vi "Delete_Zero_Columns_Rows_Resolved_Tracks-1.vi"(4 "error IN":errorcluster, 7 "[IN] Clusters for Re\nconstructed Tracks":T1) -> (0 "error OUT":errorcluster, 3 "[OUT] Clusters for Re\nconstructed Tracks":T1)   [LabVIEW 2013]
doc: "The subVI delete zero columns and rows after resolving the correspondence problems"
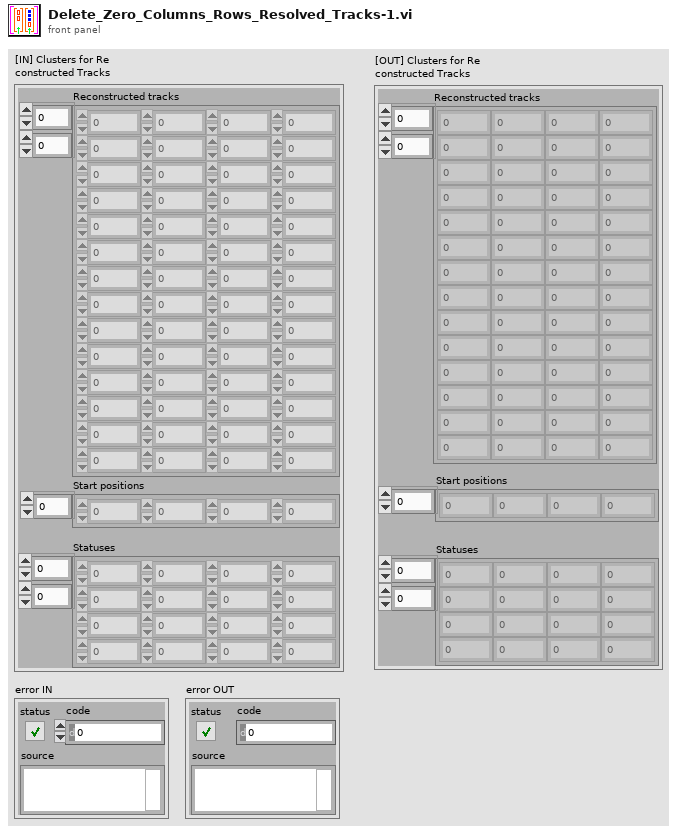
[diagram p1: front panel]
types:
  T1 = cluster{"Reconstructed tracks":dbl[][], "Start positions":i32[], "Statuses":i16[][]}
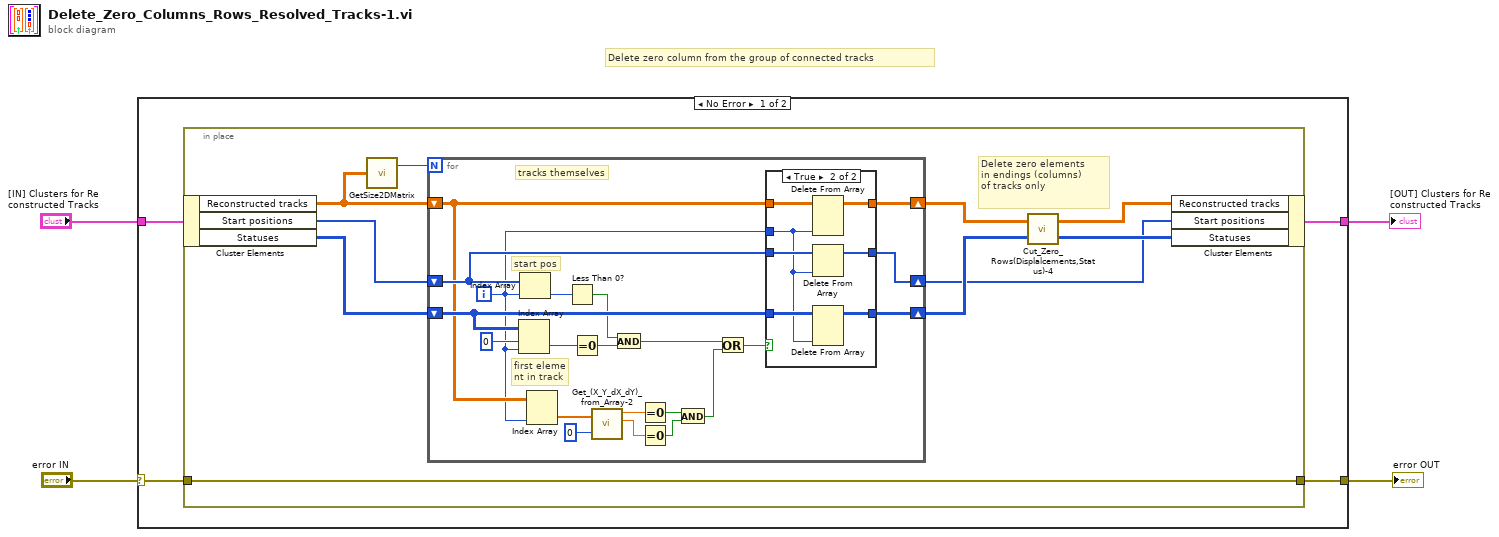
[diagram p0: block diagram]
diagram:
  # "Delete zero column from the group of connected tracks"
  n1 = case shown="No Error" "error IN" {
    selector: "error IN" -> [w6 w51]
    tunnel: "[IN] Clusters for Re\nconstructed Tracks" -> [w8 w50]
    tunnel: [w7 w50] -> w3
    tunnel: [w5 w51] -> w1
    frame No Error {
      n2 = in-place {
        in-place-border: w6 -> [w9]
        in-place-border: [w9] -> w5
        # "Delete zero elements \nin endings (columns)\nof tracks only"
        n3 = in-place-cluster #1(w8) -> ("Reconstructed tracks"=w15:dbl[][], "Start positions"=w11:i32[], "Statuses"=w10:i16[][])
        n4 = call "GetSize2DMatrix.vi"("Array IN (2D)"=w15) -> ("# Cols"=w18:i32)  [unwired: 1 out]
        n5 = for {
          N: w18 -> [_]
          shift-right: [w34] -> w17
          shift-left: w15 -> [w28]
          shift-right: [w33] -> w12
          shift-left: w11 -> [w36]
          shift-right: [w32] -> w16
          shift-left: w10 -> [w35]
          i -> [w27]
          # "tracks themselves"
          # "start pos"
          # "first eleme\nnt in track"
          n6 = Index Array(array=w35, index (row)=0, index (col)=w27) -> (element=w37:i16)
          n7 = Index Array(array=w36, index=w27) -> (element=w38:i32)
          n8 = Index Array(array=w28, index (col)=w27) -> (element=w26:dbl[])  [unwired: 1 in]
          n9 = Less Than 0?(x=w38) -> (x < 0?=w30:bool)
          n10 = Equal To 0?(x=w37) -> (x = 0?=w31:bool)
          n11 = call "Get_(X_Y_dX_dY)_from_Array-2.vi"("(X,Y,dX,dY)"=w26, "Index of Displacement"=0) -> ("X"=w24:dbl, "Y"=w23:dbl)  [unwired: 2 out]
          n12 = And(x=w30, y=w31) -> (x .and. y?=w29:bool)
          n13 = Equal To 0?(x=w24) -> (x = 0?=w22:bool)
          n14 = Equal To 0?(x=w23) -> (x = 0?=w21:bool)
          n15 = And(x=w22, y=w21) -> (x .and. y?=w19:bool)
          n16 = Or(x=w29, y=w19) -> (x .or. y?=w20:bool)
          n17 = case shown="True" w20 {
            tunnel: w28 -> [w42 w49]
            tunnel: w27 -> [_ w43]
            tunnel: w36 -> [w41 w48]
            tunnel: w35 -> [w40 w45]
            tunnel: [w42 w47] -> w34
            tunnel: [w41 w46] -> w33
            tunnel: [w40 w44] -> w32
            frame False {
            }
            frame True {
              n18 = Delete From Array(array=w49, index (col)=w43) -> (array with subset deleted=w47:dbl[][])  [unwired: 2 in, 1 out]
              n19 = Delete From Array(array=w48, index=w43) -> (array with subset deleted=w46:i32[])  [unwired: 1 in, 1 out]
              n20 = Delete From Array(array=w45, index (col)=w43) -> (array with subset deleted=w44:i16[][])  [unwired: 2 in, 1 out]
            }
          }
        }
        n21 = call "Cut_Zero_Rows(Displalcements,Status)-4.vi"("[IN] Dot matrix\nwith zero points"=w16, "[IN] (X,Y,dX,dY) \nwith zero displ"=w17) -> ("[OUT] Dot \nMatrix"=w13:i16[][], "[OUT] (X,Y,dX,dY)\nw/t zero displac"=w14:dbl[][])
        n22 = in-place-cluster #1("Reconstructed tracks"=w14, "Start positions"=w12, "Statuses"=w13) -> (w7:T1)
      }
    }
    frame Error {
    }
  }
  "error OUT" <- w1
  "[OUT] Clusters for Re\nconstructed Tracks" <- w3
